vi "ConvertDiagPacket.vi"(8 "error in (no error)":errorcluster, 10 ".NET data in":refnum<k24>, 11 "controller in":refnum<k24>) -> (0 "error out":errorcluster, 2 "LabVIEW data out":T1, 3 "controller out":refnum<k24>)   [LabVIEW 2016]
uses:
  AxisDiagPacket.ctl
  ControllerDiagPacket.ctl
  C:/user/patrick/git/Aerotech-Delay-Line/lvsrc/Aerotech-Ensemble-LabVIEW/8.2/Bin/Aerotech.Ensemble.LabVIEW.dll
  Bin/Aerotech.Ensemble.LabVIEW.dll
  C:/user/patrick/git/Aerotech-Delay-Line/lvsrc/Aerotech-Ensemble-LabVIEW/8.2/Bin/Aerotech.Ensemble.dll
  Bin/Aerotech.Ensemble.dll
panel:
  in  "ControllerDiagPacket Type":T1
  in  "AxisDiagPacket Type":T2
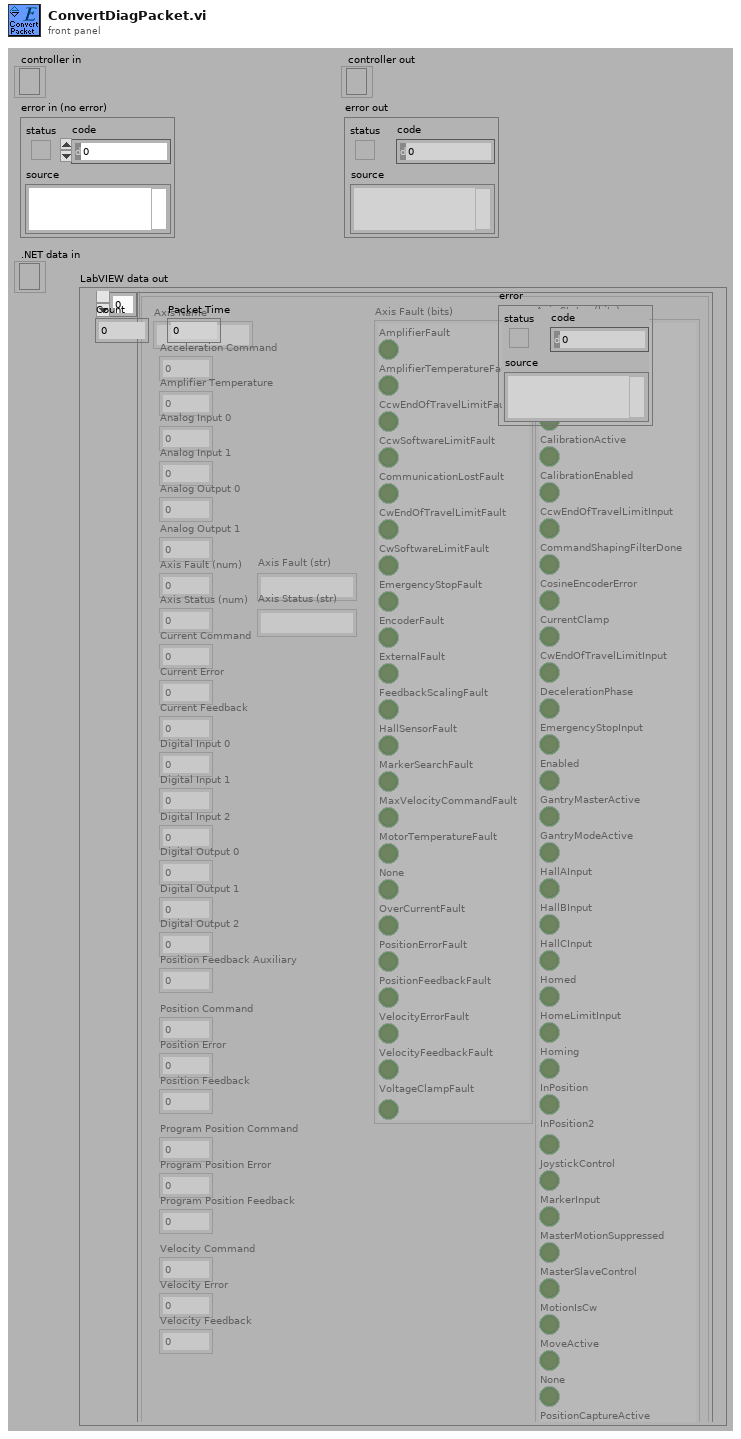
[diagram p1: front panel]
types:
  T1 = typedef "ControllerDiagPacket.ctl" = cluster{"Count":i32, "Packet Time":i64, "Axes":T2[], "error":errorcluster}
  T2 = typedef "AxisDiagPacket.ctl" = cluster{"Axis Name":string, "Acceleration Command":dbl, "Amplifier Temperature":sgl, "Analog Input 0":dbl, "Analog Input 1":dbl, "Analog Output 0":dbl, "Analog Output 1":dbl, "Axis Fault (num)":i32, "Axis Fault (str)":string, "Axis Fault (bits)":cluster{"AmplifierFault":bool, "AmplifierTemperatureFault":bool, "CcwEndOfTravelLimitFault":bool, "CcwSoftwareLimitFault":bool, "CommunicationLostFault":bool, "CwEndOfTravelLimitFault":bool, "CwSoftwareLimitFault":bool, "EmergencyStopFault":bool, "EncoderFault":bool, "ExternalFault":bool, "FeedbackScalingFault":bool, "HallSensorFault":bool, "MarkerSearchFault":bool, "MaxVelocityCommandFault":bool, "MotorTemperatureFault":bool, "None":bool, "OverCurrentFault":bool, "PositionErrorFault":bool, "PositionFeedbackFault":bool, "VelocityErrorFault":bool, "VelocityFeedbackFault":bool, "VoltageClampFault":bool}, "Axis Status (num)":i32, "Axis Status (str)":string, "Axis Status (bits)":cluster{"AccelerationPhase":bool, "AutofocusActive":bool, "BrakeOutput":bool, "CalibrationActive":bool, "CalibrationEnabled":bool, "CcwEndOfTravelLimitInput":bool, "CommandShapingFilterDone":bool, "CosineEncoderError":bool, "CurrentClamp":bool, "CwEndOfTravelLimitInput":bool, "DecelerationPhase":bool, "EmergencyStopInput":bool, "Enabled":bool, "GantryMasterActive":bool, "GantryModeActive":bool, "HallAInput":bool, "HallBInput":bool, "HallCInput":bool, "Homed":bool, "HomeLimitInput":bool, "Homing":bool, "InPosition":bool, "InPosition2":bool, "JoystickControl":bool, "MarkerInput":bool, "MasterMotionSuppressed":bool, "MasterSlaveControl":bool, "MotionIsCw":bool, "MoveActive":bool, "None":bool, "PositionCaptureActive":bool, "ServoControl":bool, "SineEncoderError":bool}, "Current Command":sgl, "Current Error":sgl, "Current Feedback":sgl, "Digital Input 0":i32, "Digital Input 1":i32, "Digital Input 2":i32, "Digital Output 0":i32, "Digital Output 1":i32, "Digital Output 2":i32, "Position Feedback Auxiliary":dbl, "Position Command":dbl, "Position Error":dbl, "Position Feedback":dbl, "Program Position Command":dbl, "Program Position Error":dbl, "Program Position Feedback":dbl, "Velocity Command":dbl, "Velocity Error":dbl, "Velocity Feedback":dbl}
  T3 = cluster{"AccelerationPhase":bool, "AutofocusActive":bool, "BrakeOutput":bool, "CalibrationActive":bool, "CalibrationEnabled":bool, "CcwEndOfTravelLimitInput":bool, "CommandShapingFilterDone":bool, "CosineEncoderError":bool, "CurrentClamp":bool, "CwEndOfTravelLimitInput":bool, "DecelerationPhase":bool, "EmergencyStopInput":bool, "Enabled":bool, "GantryMasterActive":bool, "GantryModeActive":bool, "HallAInput":bool, "HallBInput":bool, "HallCInput":bool, "Homed":bool, "HomeLimitInput":bool, "Homing":bool, "InPosition":bool, "InPosition2":bool, "JoystickControl":bool, "MarkerInput":bool, "MasterMotionSuppressed":bool, "MasterSlaveControl":bool, "MotionIsCw":bool, "MoveActive":bool, "None":bool, "PositionCaptureActive":bool, "ServoControl":bool, "SineEncoderError":bool}
  T4 = cluster{"AmplifierFault":bool, "AmplifierTemperatureFault":bool, "CcwEndOfTravelLimitFault":bool, "CcwSoftwareLimitFault":bool, "CommunicationLostFault":bool, "CwEndOfTravelLimitFault":bool, "CwSoftwareLimitFault":bool, "EmergencyStopFault":bool, "EncoderFault":bool, "ExternalFault":bool, "FeedbackScalingFault":bool, "HallSensorFault":bool, "MarkerSearchFault":bool, "MaxVelocityCommandFault":bool, "MotorTemperatureFault":bool, "None":bool, "OverCurrentFault":bool, "PositionErrorFault":bool, "PositionFeedbackFault":bool, "VelocityErrorFault":bool, "VelocityFeedbackFault":bool, "VoltageClampFault":bool}
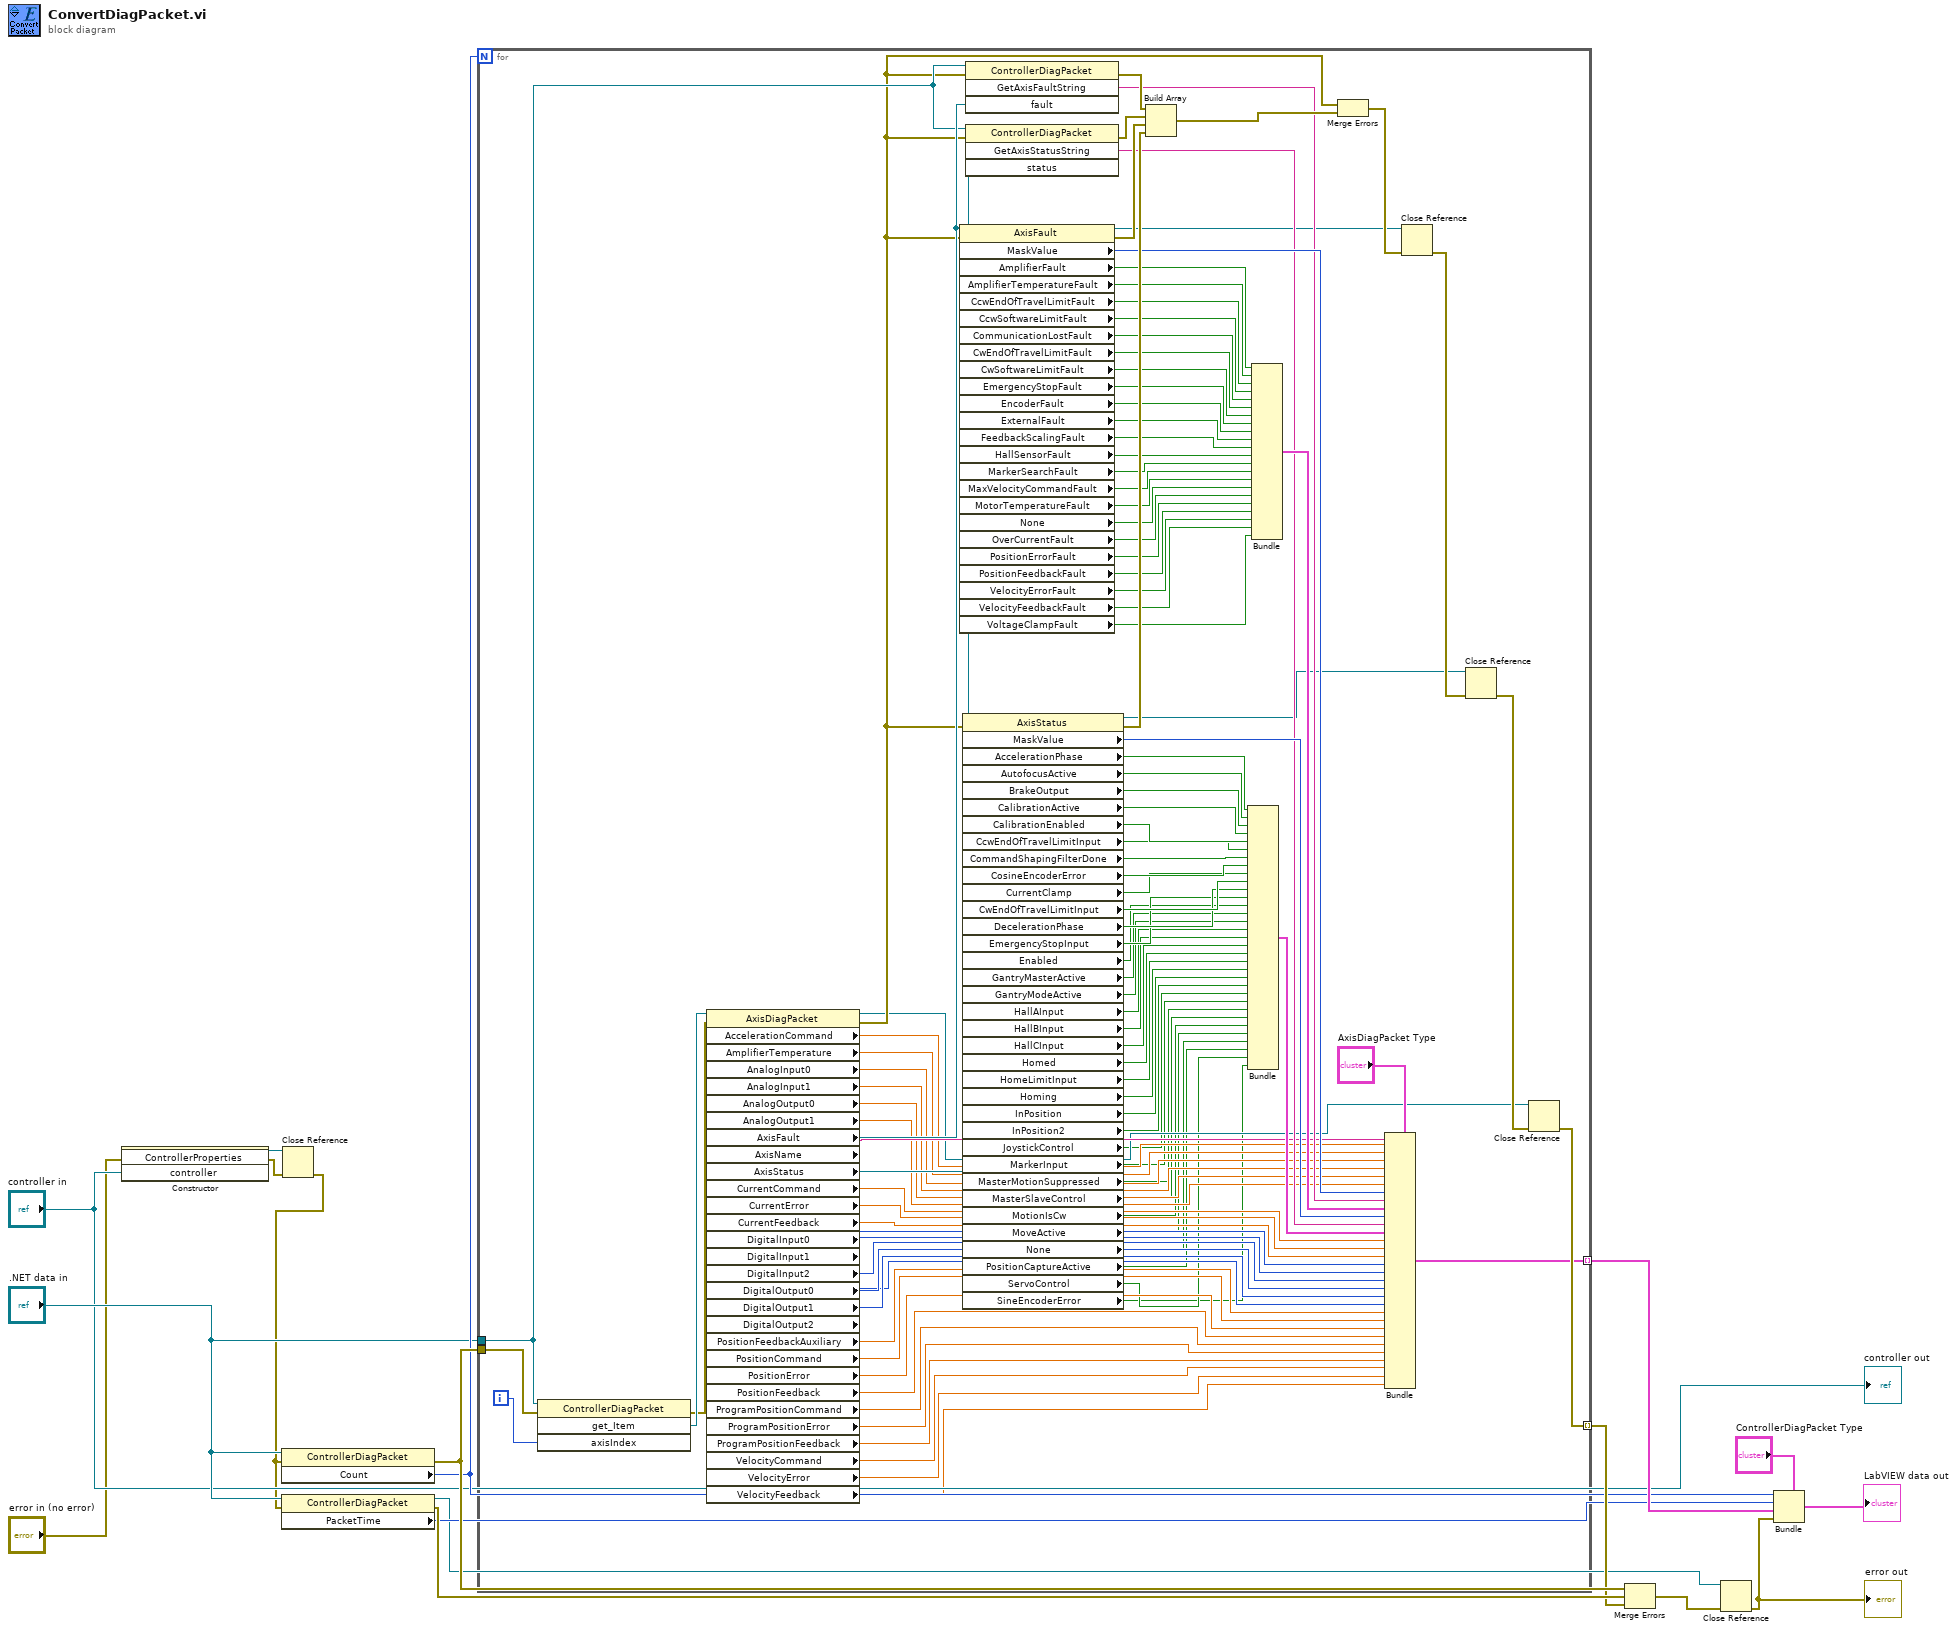
[diagram p0: block diagram]
diagram:
  n1 = constructor class="ControllerProperties"(error in="error in (no error)", "controller"="controller in") -> (reference out=w3:refnum<k24>, error out=w1:errorcluster)  [unwired: 2 in, 2 out]
  n2 = Close Reference(reference=w3, error in (no error)=w1) -> (error out=w2:errorcluster)
  n3 = property class="ControllerDiagPacket"(reference=".NET data in", error in=w2) -> (error out=w16:errorcluster, "Count"=w12:i32)  [unwired: 1 out]
  n4 = property class="ControllerDiagPacket"(reference=".NET data in", error in=w2) -> (reference out=w6:refnum<k24>, error out=w17:errorcluster, "PacketTime"=w13:i64)
  n5 = for {
    N: w12 -> [_]
    tunnel: [w90] -> w14 mode=indexing
    tunnel: w16 -> [w125]
    tunnel: ".NET data in" -> [w114]
    tunnel: [w96] -> w15 mode=indexing
    i -> [w126]
    n6 = invoke class="ControllerDiagPacket" method="get_Item"(reference=w114, error in=w125, "axisIndex"=w126) -> (error out=w123:errorcluster, "get_Item"=w124:refnum<k24>)  [unwired: 1 in, 2 out]
    n7 = property class="AxisDiagPacket"(reference=w124, error in=w123) -> (reference out=w61:refnum<k24>, error out=w68:errorcluster, "AccelerationCommand"=w67:dbl, "AmplifierTemperature"=w66:sgl, "AnalogInput0"=w65:dbl, "AnalogInput1"=w64:dbl, "AnalogOutput0"=w63:dbl, "AnalogOutput1"=w62:dbl, "AxisFault"=w116:refnum<k24>, "AxisName"=w78:string, "AxisStatus"=w115:refnum<k24>, "CurrentCommand"=w88:sgl, "CurrentError"=w87:sgl, "CurrentFeedback"=w86:sgl, "DigitalInput0"=w85:i32, "DigitalInput1"=w84:i32, "DigitalInput2"=w83:i32, "DigitalOutput0"=w82:i32, "DigitalOutput1"=w81:i32, "DigitalOutput2"=w80:i32, "PositionFeedbackAuxiliary"=w79:dbl, "PositionCommand"=w77:dbl, "PositionError"=w76:dbl, "PositionFeedback"=w75:dbl, "ProgramPositionCommand"=w74:dbl, "ProgramPositionError"=w73:dbl, "ProgramPositionFeedback"=w72:dbl, "VelocityCommand"=w71:dbl, "VelocityError"=w70:dbl, "VelocityFeedback"=w69:dbl)
    n8 = property class="AxisFault"(reference=w116, error in=w68) -> (reference out=w92:refnum<k24>, error out=w119:errorcluster, "MaskValue"=w117:i32, "AmplifierFault"=w41:bool, "AmplifierTemperatureFault"=w40:bool, "CcwEndOfTravelLimitFault"=w39:bool, "CcwSoftwareLimitFault"=w38:bool, "CommunicationLostFault"=w37:bool, "CwEndOfTravelLimitFault"=w36:bool, "CwSoftwareLimitFault"=w35:bool, "EmergencyStopFault"=w34:bool, "EncoderFault"=w33:bool, "ExternalFault"=w32:bool, "FeedbackScalingFault"=w31:bool, "HallSensorFault"=w30:bool, "MarkerSearchFault"=w29:bool, "MaxVelocityCommandFault"=w28:bool, "MotorTemperatureFault"=w27:bool, "None"=w26:bool, "OverCurrentFault"=w25:bool, "PositionErrorFault"=w24:bool, "PositionFeedbackFault"=w23:bool, "VelocityErrorFault"=w22:bool, "VelocityFeedbackFault"=w21:bool, "VoltageClampFault"=w18:bool)
    n9 = property class="AxisStatus"(reference=w115, error in=w68) -> (reference out=w91:refnum<k24>, error out=w118:errorcluster, "MaskValue"=w99:i32, "AccelerationPhase"=w113:bool, "AutofocusActive"=w112:bool, "BrakeOutput"=w111:bool, "CalibrationActive"=w110:bool, "CalibrationEnabled"=w109:bool, "CcwEndOfTravelLimitInput"=w108:bool, "CommandShapingFilterDone"=w107:bool, "CosineEncoderError"=w106:bool, "CurrentClamp"=w105:bool, "CwEndOfTravelLimitInput"=w104:bool, "DecelerationPhase"=w103:bool, "EmergencyStopInput"=w102:bool, "Enabled"=w60:bool, "GantryMasterActive"=w59:bool, "GantryModeActive"=w58:bool, "HallAInput"=w57:bool, "HallBInput"=w56:bool, "HallCInput"=w55:bool, "Homed"=w54:bool, "HomeLimitInput"=w53:bool, "Homing"=w52:bool, "InPosition"=w51:bool, "InPosition2"=w50:bool, "JoystickControl"=w49:bool, "MarkerInput"=w48:bool, "MasterMotionSuppressed"=w47:bool, "MasterSlaveControl"=w46:bool, "MotionIsCw"=w45:bool, "MoveActive"=w44:bool, "None"=w43:bool, "PositionCaptureActive"=w42:bool, "ServoControl"=w20:bool, "SineEncoderError"=w19:bool)
    n10 = invoke class="ControllerDiagPacket" method="GetAxisFaultString"(reference=w114, error in=w68, "fault"=w116) -> (error out=w122:errorcluster, "GetAxisFaultString"=w101:string)  [unwired: 1 in, 2 out]
    n11 = invoke class="ControllerDiagPacket" method="GetAxisStatusString"(reference=w114, error in=w68, "status"=w115) -> (error out=w120:errorcluster, "GetAxisStatusString"=w98:string)  [unwired: 1 in, 2 out]
    n12 = Build Array(w122, w120, w119, w118) -> (w121:errorcluster[])
    n13 = Bundle("AccelerationPhase"=w113, "AutofocusActive"=w112, "BrakeOutput"=w111, "CalibrationActive"=w110, "CalibrationEnabled"=w109, "CcwEndOfTravelLimitInput"=w108, "CommandShapingFilterDone"=w107, "CosineEncoderError"=w106, "CurrentClamp"=w105, "CwEndOfTravelLimitInput"=w104, "DecelerationPhase"=w103, "EmergencyStopInput"=w102, "Enabled"=w60, "GantryMasterActive"=w59, "GantryModeActive"=w58, "HallAInput"=w57, "HallBInput"=w56, "HallCInput"=w55, "Homed"=w54, "HomeLimitInput"=w53, "Homing"=w52, "InPosition"=w51, "InPosition2"=w50, "JoystickControl"=w49, "MarkerInput"=w48, "MasterMotionSuppressed"=w47, "MasterSlaveControl"=w46, "MotionIsCw"=w45, "MoveActive"=w44, "None"=w43, "PositionCaptureActive"=w42, "ServoControl"=w20, "SineEncoderError"=w19) -> (w97:T3)  [unwired: 1 in]
    n14 = Bundle("AmplifierFault"=w41, "AmplifierTemperatureFault"=w40, "CcwEndOfTravelLimitFault"=w39, "CcwSoftwareLimitFault"=w38, "CommunicationLostFault"=w37, "CwEndOfTravelLimitFault"=w36, "CwSoftwareLimitFault"=w35, "EmergencyStopFault"=w34, "EncoderFault"=w33, "ExternalFault"=w32, "FeedbackScalingFault"=w31, "HallSensorFault"=w30, "MarkerSearchFault"=w29, "MaxVelocityCommandFault"=w28, "MotorTemperatureFault"=w27, "None"=w26, "OverCurrentFault"=w25, "PositionErrorFault"=w24, "PositionFeedbackFault"=w23, "VelocityErrorFault"=w22, "VelocityFeedbackFault"=w21, "VoltageClampFault"=w18) -> (w100:T4)  [unwired: 1 in]
    n15 = Merge Errors(w68, w121) -> (w93:errorcluster)
    n16 = Bundle(cluster="AxisDiagPacket Type", "Axis Name"=w78, "Acceleration Command"=w67, "Amplifier Temperature"=w66, "Analog Input 0"=w65, "Analog Input 1"=w64, "Analog Output 0"=w63, "Analog Output 1"=w62, "Axis Fault (num)"=w117, "Axis Fault (str)"=w101, "Axis Fault (bits)"=w100, "Axis Status (num)"=w99, "Axis Status (str)"=w98, "Axis Status (bits)"=w97, "Current Command"=w88, "Current Error"=w87, "Current Feedback"=w86, "Digital Input 0"=w85, "Digital Input 1"=w84, "Digital Input 2"=w83, "Digital Output 0"=w82, "Digital Output 1"=w81, "Digital Output 2"=w80, "Position Feedback Auxiliary"=w79, "Position Command"=w77, "Position Error"=w76, "Position Feedback"=w75, "Program Position Command"=w74, "Program Position Error"=w73, "Program Position Feedback"=w72, "Velocity Command"=w71, "Velocity Error"=w70, "Velocity Feedback"=w69) -> (w90:T2)
    n17 = Close Reference(reference=w92, error in (no error)=w93) -> (error out=w94:errorcluster)
    n18 = Close Reference(reference=w91, error in (no error)=w94) -> (error out=w95:errorcluster)
    n19 = Close Reference(reference=w61, error in (no error)=w95) -> (error out=w96:errorcluster)
  }
  n20 = Merge Errors(w16, w17, w15) -> (w8:errorcluster)
  n21 = Close Reference(reference=w6, error in (no error)=w8) -> (error out=w7:errorcluster)
  "error out" <- w7
  n22 = Bundle(cluster="ControllerDiagPacket Type", "Count"=w12, "Packet Time"=w13, "Axes"=w14, "error"=w7) -> (→"LabVIEW data out":T1)
  "controller out" <- "controller in"
